vi "Set Parent Values from Template.vi"(0 "template configuration":refnum<class "SV Signal.lvclass">, 2 "signal configuration in":refnum<class "SV Signal.lvclass">, 7 "error in (no error)":errorcluster) -> (4 "signal configuration out":refnum<class "SV Signal.lvclass">, 6 "template used?":bool, 8 "error out":errorcluster)   [LabVIEW 2017, in "SV Signal.lvclass"]
uses:
  <vilib>/addons/_NISVFA/_Generation/Signal Generation/SV Signal/SV Signal.lvclass
  <vilib>/addons/_NISVFA/_Generation/Signal Generation/SV Signal/SV Signal.lvclass/SV Signal.ctl
  <vilib>/addons/_NISVFA/_Generation/Signal Generation/SV Signal/sv_System Timing Model.ctl
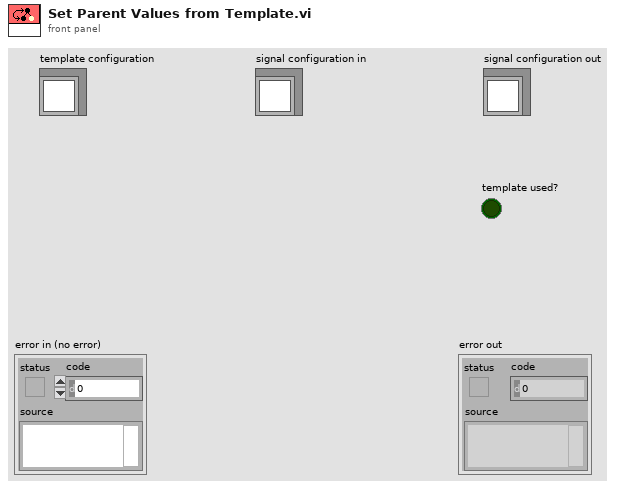
[diagram p1: front panel]
types:
  T1 = typedef "SV Signal.lvclass/sv_System Timing Model.ctl" = i64
  T2 = cluster{"profile":enum16{"Linear", "Half cosine"}, "durations [s]":cluster{"ramp-up":dbl, "transition":dbl, "ramp-down":dbl}}
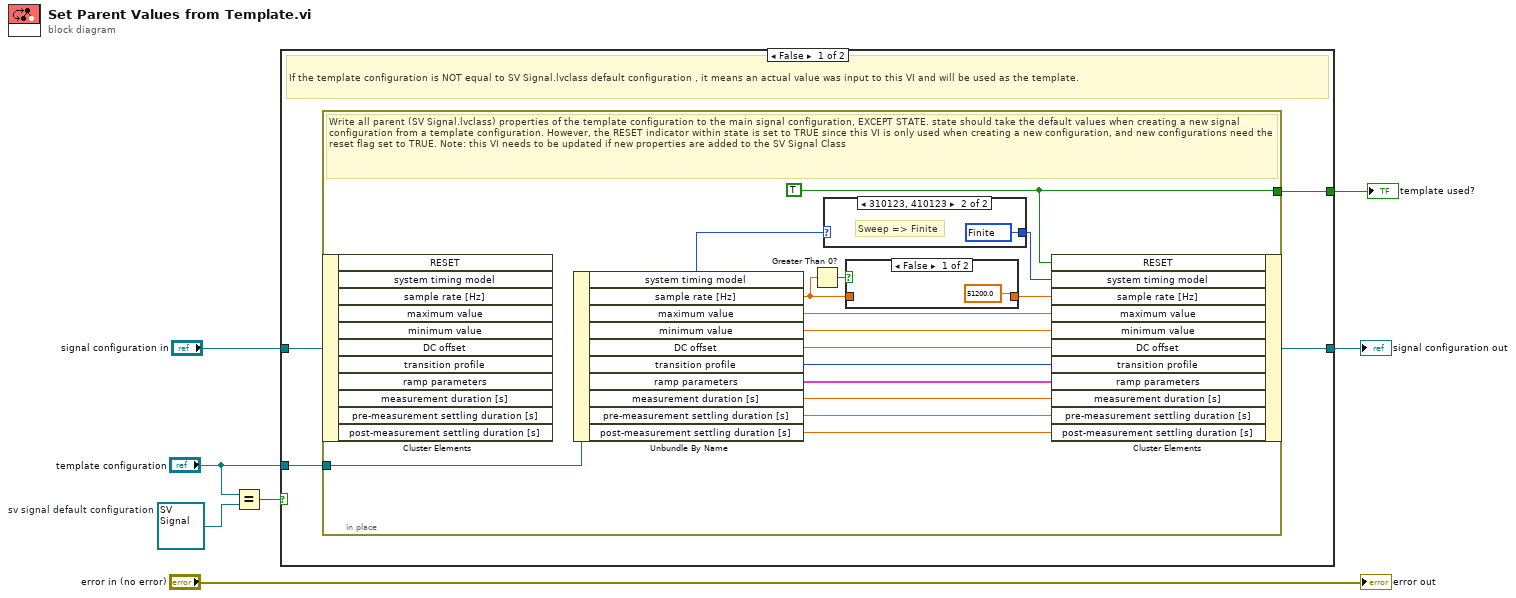
[diagram p0: block diagram]
diagram:
  w4 = refnum<class "SV Signal.lvclass"> refnum  # sv signal default configuration
  n1 = Equal?(x="template configuration", y=w4) -> (x = y?=w1:bool)
  n2 = case shown="False" w1 {
    tunnel: "signal configuration in" -> [w11 w31]
    tunnel: [w10 w31] -> w6
    tunnel: "template configuration" -> [w9 _]
    tunnel: [w8 _] -> w5
    frame False {
      # "If the template configuration is NOT equal to SV Signal.lvclass default configuration , it means an actual value was input to this VI and will be used as the template."
      n3 = in-place {
        in-place-border: w9 -> [w26]
        in-place-border: [w18] -> w8
        w18 = TRUE ("state.RESET")
        # "Write all parent (SV Signal.lvclass) properties of the template configuration to the main signal configuration, EXCEPT STATE. state should take the default values when creating a new signal configuration from a template configuration. However, the RESET indicator within state is set to TRUE since this VI is only used when creating a new configuration, and new configurations need the reset flag set to TRUE. Note: this VI needs to be updated if new properties are added to the SV Signal Class"
        n4 = in-place-cluster #1(w11) -> ()  [unwired: 11 out]
        n5 = Unbundle By Name(w26) -> ("system timing model"=w17:T1, "sample rate [Hz]"=w13:dbl, "maximum value"=w25:dbl, "minimum value"=w24:dbl, "DC offset"=w23:dbl, "transition profile"=w22:enum16{"Immediate", "Next optimum", "Ramp"}, "ramp parameters"=w21:T2, "measurement duration [s]"=w20:dbl, "pre-measurement settling duration [s]"=w19:dbl, "post-measurement settling duration [s]"=w15:dbl)
        n6 = Greater Than 0?(x=w13) -> (x > 0?=w14:bool)
        n7 = case shown="310123, 410123" w17 {
          selector: w17 -> [w29 _]
          tunnel: [w29 w30] -> w16
          frame Default {
          }
          frame 310123, 410123 {
            w30 = T1 10178 items=["Finite"=10178, "-"=-1, "Continuous"=10123, "-"=-2, "Settled"=110123, "Averaged"=210123, "Discrete Sweep"=310123, "Continuous Sweep"=410123] ("system timing model")
            # "Sweep => Finite"
          }
        }
        n8 = case shown="False" w14 {
          tunnel: w13 -> [_ w28]
          tunnel: [51200.0 ("sample rate [Hz]") w28] -> w12
          frame False {
          }
          frame True {
          }
        }
        n9 = in-place-cluster #1("RESET"=w18, "system timing model"=w16, "sample rate [Hz]"=w12, "maximum value"=w25, "minimum value"=w24, "DC offset"=w23, "transition profile"=w22, "ramp parameters"=w21, "measurement duration [s]"=w20, "pre-measurement settling duration [s]"=w19, "post-measurement settling duration [s]"=w15) -> (w10:refnum<class "SV Signal.lvclass">)
      }
    }
    frame True {
      # "If template is equal to the SV Signal.lvclass default configuration, then we assume nothing was wired to the template configuration, so there is no need to apply the template. Only a child of SV signal indicates an actual template configuration was wired to the control"
    }
  }
  "signal configuration out" <- w6
  "template used?" <- w5
  "error out" <- "error in (no error)"
